vi "initialize.vi"(8 "error in (no error)":errorcluster, 10 "Distance Threshold":dbl, 11 "Desired UTM Location":T1) -> (0 "error out":errorcluster, 3 "Drive Mission":refnum<class "Drive.lvclass">)   [LabVIEW 2011, in "Drive.lvclass"]
uses:
  Drive.lvclass
  2-RIO/2 Typedefs/UTM Location.ctl
  Drive.lvclass/Drive.ctl
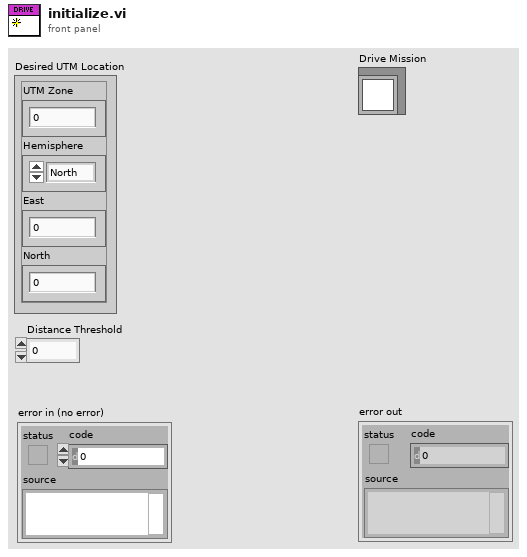
[diagram p1: front panel]
types:
  T1 = typedef "UTM Location.ctl" = cluster{"UTM Zone":dbl, "Hemisphere":enum16{"North", "South"}, "East":dbl, "North":dbl}
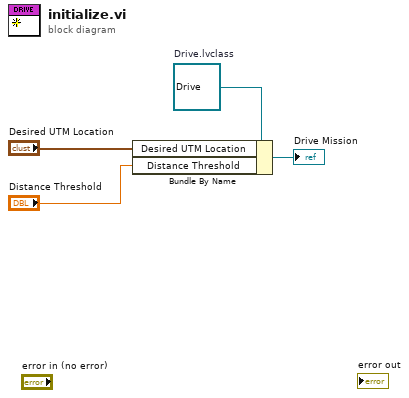
[diagram p0: block diagram]
diagram:
  w4 = refnum<class "Drive.lvclass"> refnum  # Drive.lvclass
  n1 = Bundle By Name(cluster=w4, "Desired UTM Location"="Desired UTM Location", "Distance Threshold"="Distance Threshold") -> (→"Drive Mission":refnum<class "Drive.lvclass">)
